vi "hw5_2_(2).vi"() -> ()   [LabVIEW 2014]
panel:
  in  "stop":bool
  out "Result":string
  in  "Calculator":T1
  # "每次只能做兩個值的運算\nex 1+2+3+4=10\n-> 1+2=3\n      3+3=6\n      6+4=10"
  # "助教說可以這樣～"
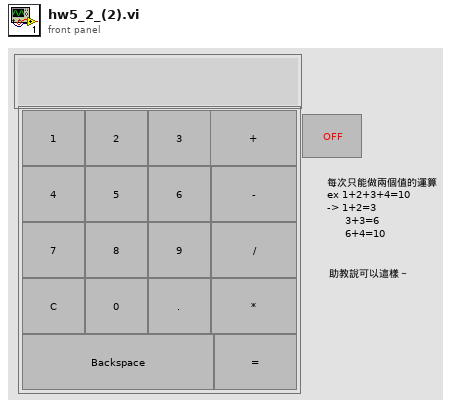
[diagram p1: front panel]
types:
  T1 = cluster{"2":bool, "3":bool, "4":bool, "5":bool, "6":bool, "7":bool, "8":bool, "9":bool, "*":bool, "=":bool, "backspace":bool, "0":bool, ".":bool, "C":bool, "/":bool, "-":bool, "+":bool, "1":bool}
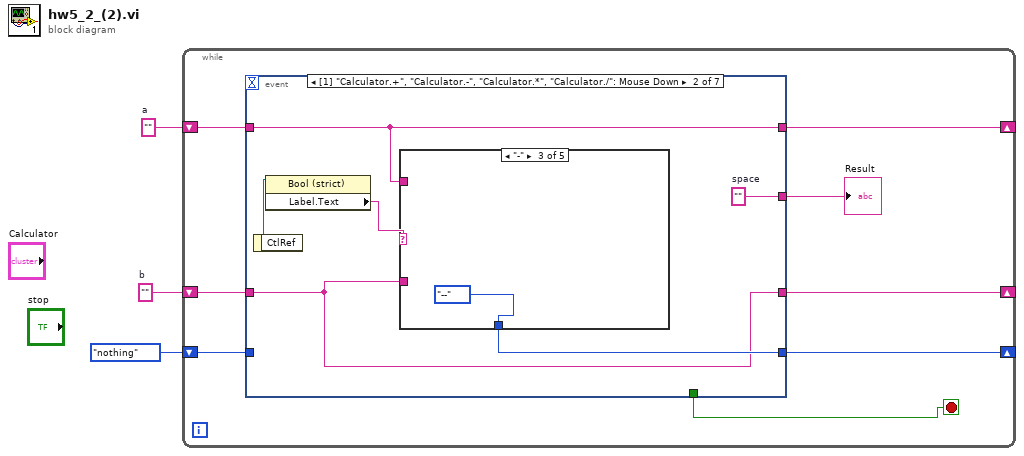
[diagram p0: block diagram]
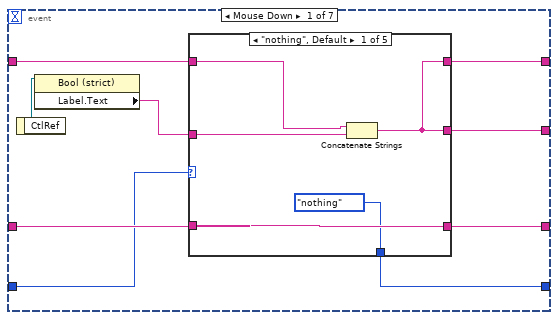
[diagram p2: hidden frame]
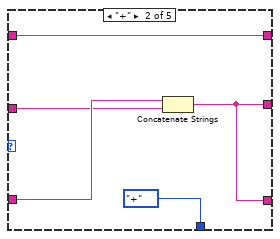
[diagram p3: hidden frame]
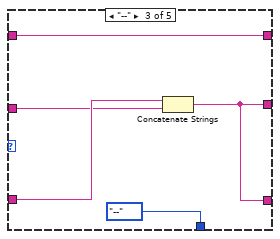
[diagram p4: hidden frame]
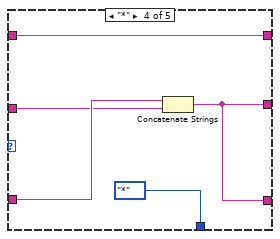
[diagram p5: hidden frame]
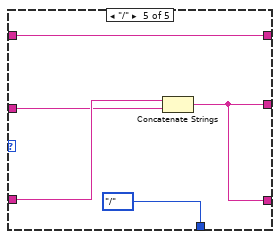
[diagram p6: hidden frame]
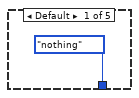
[diagram p7: hidden frame]
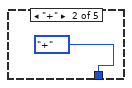
[diagram p8: hidden frame]
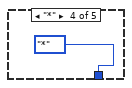
[diagram p9: hidden frame]
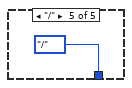
[diagram p10: hidden frame]
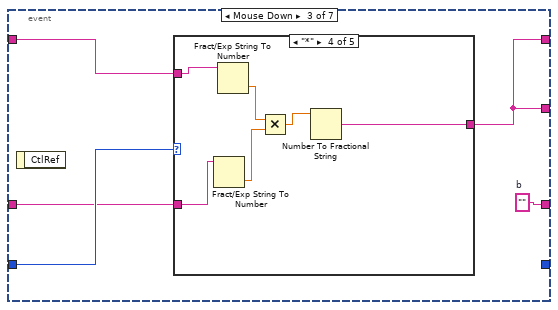
[diagram p11: hidden frame]
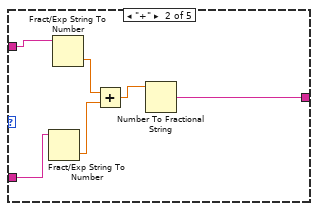
[diagram p13: hidden frame]
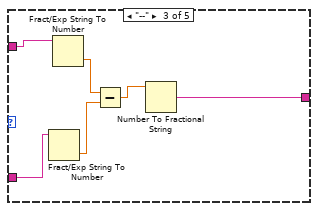
[diagram p14: hidden frame]
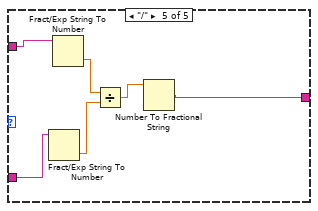
[diagram p15: hidden frame]
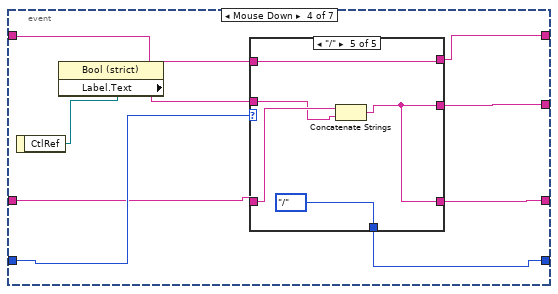
[diagram p16: hidden frame]
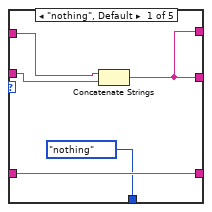
[diagram p17: hidden frame]
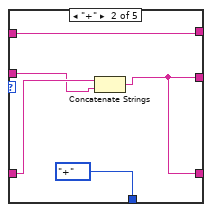
[diagram p18: hidden frame]
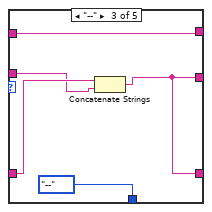
[diagram p19: hidden frame]
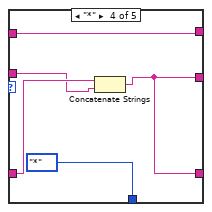
[diagram p20: hidden frame]
diagram:
  w1 = ""  # b
  w3 = ""  # a
  n1 = while {
    shift-right: [w5] -> _
    shift-left: w3 -> [w11]
    shift-right: [w10] -> _
    shift-left: enum16{"nothing", "+", "--", "*", "/"}."nothing" -> [w7]
    shift-right: [w8] -> _
    shift-left: w1 -> [w9]
    stop <- w4 stop-if-true
    n2 = event shown="[1] \"Calculator.+\", \"Calculator.-\", \"Calculator.*\", \"Calculator./\": Mouse Down" {
      selector: _ -> [_ _ _ _ _ _ _]
      dyn-events: _ -> [_ _ _ _ _ _ _]
      timeout: _ -> [_ _ _ _ _ _ _]
      tunnel: w11 -> [w19 w47 w59 w90 w123 _ _]
      tunnel: [w12 w50 _ w91 w127 _ _] -> w10
      tunnel: w9 -> [w17 w46 w60 w87 w122 _ _]
      tunnel: [w15 w46 w57 w92 w126 w158 _] -> w8
      tunnel: w7 -> [w13 _ w61 w88 w121 _ _]
      tunnel: [w16 w48 w58 w93 w125 w158 _] -> w6
      tunnel: [w14 w47 w58 w94 w124 w158 _] -> w5
      tunnel: [_ _ _ _ _ _ TRUE] -> w4
      event "Calculator.1", "Calculator.2", "Calculator.3", "Calculator.4", "Calculator.5", "Calculator.6", "Calculator.7", "Calculator.8", "Calculator.9", "Calculator.0": Mouse Down {
        n3 = event-data() -> ("CtlRef"=w20:refnum<vi>)  [unwired: 1 in]
        n4 = property class="Bool (strict)"(reference=w20) -> ("Label.Text"=w18:string)  [unwired: 1 in, 2 out]
        n5 = case shown="\"nothing\", Default" w13 {
          tunnel: w19 -> [w24 w29 w34 w39 w44]
          tunnel: w18 -> [w22 w26 w31 w36 w41]
          tunnel: [w21 w27 w32 w37 w43] -> w16
          tunnel: w17 -> [w25 w30 w35 w40 w45]
          tunnel: [w25 w27 w32 w37 w43] -> w15
          tunnel: [w21 w29 w34 w39 w44] -> w14
          tunnel: [enum16{"nothing", "+", "--", "*", "/"}."nothing" enum16{"nothing", "+", "--", "*", "/"}."+" enum16{"nothing", "+", "--", "*", "/"}."--" enum16{"nothing", "+", "--", "*", "/"}."*" enum16{"nothing", "+", "--", "*", "/"}."/"] -> w12
          frame "nothing", Default {
            n6 = Concatenate Strings(w24, w22) -> (w21:string)
          }
          frame "+" {
            n7 = Concatenate Strings(w30, w26) -> (w27:string)
          }
          frame "--" {
            n8 = Concatenate Strings(w35, w31) -> (w32:string)
          }
          frame "*" {
            n9 = Concatenate Strings(w40, w36) -> (w37:string)
          }
          frame "/" {
            n10 = Concatenate Strings(w45, w41) -> (w43:string)
          }
        }
      }
      event "Calculator.+", "Calculator.-", "Calculator.*", "Calculator./": Mouse Down {
        w48 = ""  # space
        n11 = event-data() -> ("CtlRef"=w51:refnum<vi>)  [unwired: 1 in]
        n12 = property class="Bool (strict)"(reference=w51) -> ("Label.Text"=w49:string)  [unwired: 1 in, 2 out]
        n13 = case shown="\"-\"" w49 {
          tunnel: [enum16{"nothing", "+", "--", "*", "/"}."nothing" enum16{"nothing", "+", "--", "*", "/"}."+" enum16{"nothing", "+", "--", "*", "/"}."--" enum16{"nothing", "+", "--", "*", "/"}."*" enum16{"nothing", "+", "--", "*", "/"}."/"] -> w50
          tunnel: w47 -> [_ _ _ _ _]
          tunnel: w46 -> [_ _ _ _ _]
          frame Default {
          }
          frame "+" {
          }
          frame "-" {
          }
          frame "*" {
          }
          frame "/" {
          }
        }
      }
      event "Calculator.=": Mouse Down {
        w57 = ""  # b
        n14 = event-data() -> ()  [unwired: 1 in, 1 out]
        n15 = case shown="\"*\"" w61 {
          tunnel: w60 -> [_ w65 w71 w77 w84]
          tunnel: [w62 w64 w70 w76 w82] -> w58
          tunnel: w59 -> [w62 w63 w69 w75 w81]
          frame "nothing", Default {
          }
          frame "+" {
            n16 = Fract/Exp String To Number(string=w65) -> (number=w67:dbl)  [unwired: 3 in, 1 out]
            n17 = Fract/Exp String To Number(string=w63) -> (number=w68:dbl)  [unwired: 3 in, 1 out]
            n18 = Add(x=w68, y=w67) -> (x+y=w66:dbl)
            n19 = Number To Fractional String(number=w66) -> (F-format string=w64:string)  [unwired: 3 in]
          }
          frame "--" {
            n20 = Fract/Exp String To Number(string=w71) -> (number=w73:dbl)  [unwired: 3 in, 1 out]
            n21 = Fract/Exp String To Number(string=w69) -> (number=w74:dbl)  [unwired: 3 in, 1 out]
            n22 = Subtract(x=w74, y=w73) -> (x-y=w72:dbl)
            n23 = Number To Fractional String(number=w72) -> (F-format string=w70:string)  [unwired: 3 in]
          }
          frame "*" {
            n24 = Fract/Exp String To Number(string=w77) -> (number=w79:dbl)  [unwired: 3 in, 1 out]
            n25 = Fract/Exp String To Number(string=w75) -> (number=w80:dbl)  [unwired: 3 in, 1 out]
            n26 = Multiply(x=w80, y=w79) -> (x*y=w78:dbl)
            n27 = Number To Fractional String(number=w78) -> (F-format string=w76:string)  [unwired: 3 in]
          }
          frame "/" {
            n28 = Fract/Exp String To Number(string=w84) -> (number=w85:dbl)  [unwired: 3 in, 1 out]
            n29 = Fract/Exp String To Number(string=w81) -> (number=w86:dbl)  [unwired: 3 in, 1 out]
            n30 = Divide(x=w86, y=w85) -> (x/y=w83:dbl)
            n31 = Number To Fractional String(number=w83) -> (F-format string=w82:string)  [unwired: 3 in]
          }
        }
      }
      event "Calculator..": Mouse Down {
        n32 = event-data() -> ("CtlRef"=w89:refnum<vi>)  [unwired: 1 in]
        n33 = property class="Bool (strict)"(reference=w89) -> ("Label.Text"=w95:string)  [unwired: 1 in, 2 out]
        n34 = case shown="\"/\"" w88 {
          tunnel: w90 -> [w98 w103 w108 w113 w118]
          tunnel: w95 -> [w100 w104 w109 w114 w119]
          tunnel: [w97 w102 w107 w112 w117] -> w93
          tunnel: w87 -> [w99 w105 w110 w115 w120]
          tunnel: [w99 w102 w107 w112 w117] -> w92
          tunnel: [w97 w103 w108 w113 w118] -> w94
          tunnel: [enum16{"nothing", "+", "--", "*", "/"}."nothing" enum16{"nothing", "+", "--", "*", "/"}."+" enum16{"nothing", "+", "--", "*", "/"}."--" enum16{"nothing", "+", "--", "*", "/"}."*" enum16{"nothing", "+", "--", "*", "/"}."/"] -> w91
          frame "nothing", Default {
            n35 = Concatenate Strings(w98, w100) -> (w97:string)
          }
          frame "+" {
            n36 = Concatenate Strings(w105, w104) -> (w102:string)
          }
          frame "--" {
            n37 = Concatenate Strings(w110, w109) -> (w107:string)
          }
          frame "*" {
            n38 = Concatenate Strings(w115, w114) -> (w112:string)
          }
          frame "/" {
            n39 = Concatenate Strings(w120, w119) -> (w117:string)
          }
        }
      }
      event "Calculator.backspace": Mouse Down {
        n40 = event-data() -> ()  [unwired: 1 in, 1 out]
        n41 = case shown="\"nothing\", Default" w121 {
          tunnel: w123 -> [w130 w137 w143 w149 w155]
          tunnel: [w132 w135 w141 w147 w153] -> w125
          tunnel: w122 -> [w133 w136 w142 w148 w154]
          tunnel: [w133 w135 w141 w147 w153] -> w126
          tunnel: [w132 w137 w143 w149 w155] -> w124
          tunnel: [enum16{"nothing", "+", "--", "*", "/"}."nothing" enum16{"nothing", "+", "--", "*", "/"}."+" enum16{"nothing", "+", "--", "*", "/"}."--" enum16{"nothing", "+", "--", "*", "/"}."*" enum16{"nothing", "+", "--", "*", "/"}."/"] -> w127
          frame "nothing", Default {
            n42 = String Length(string=w130) -> (length=w129:i32)
            n43 = Decrement(x=w129) -> (x-1=w128:i32)
            n44 = String Subset(string=w130, length (rest)=w128) -> (substring=w132:string)  [unwired: 1 in]
          }
          frame "+" {
            n45 = String Length(string=w136) -> (length=w138:i32)
            n46 = Decrement(x=w138) -> (x-1=w134:i32)
            n47 = String Subset(string=w136, length (rest)=w134) -> (substring=w135:string)  [unwired: 1 in]
          }
          frame "--" {
            n48 = String Length(string=w142) -> (length=w144:i32)
            n49 = Decrement(x=w144) -> (x-1=w140:i32)
            n50 = String Subset(string=w142, length (rest)=w140) -> (substring=w141:string)  [unwired: 1 in]
          }
          frame "*" {
            n51 = String Length(string=w148) -> (length=w150:i32)
            n52 = Decrement(x=w150) -> (x-1=w146:i32)
            n53 = String Subset(string=w148, length (rest)=w146) -> (substring=w147:string)  [unwired: 1 in]
          }
          frame "/" {
            n54 = String Length(string=w154) -> (length=w156:i32)
            n55 = Decrement(x=w156) -> (x-1=w152:i32)
            n56 = String Subset(string=w154, length (rest)=w152) -> (substring=w153:string)  [unwired: 1 in]
          }
        }
      }
      event "Calculator.C": Mouse Down {
        w158 = ""  # null
        n57 = event-data() -> ()  [unwired: 1 in, 8 out]
      }
      event "stop": Mouse Down {
        n58 = event-data() -> ()  [unwired: 1 in, 8 out]
      }
    }
    "Result" <- w6
  }
